vi "α粒子的能量损失.vi"() -> ()   [LabVIEW 2014]
panel:
  out "当前放射源":string(combo) caption="放射源"
  in  "放大倍数":dbl min=0.0 max=2.0
  in  "按钮_提示":bool caption="提示"
  in  "按钮_退出":bool caption="退出"
  out "是否真空":bool
  out "信号输出":bool
  out "是否放置吸收片":bool
  out "是否放置放射源":bool
  in  "数组_电压数据名":string[](array[string])
  in  "选项卡_实验内容":T1(tab)
  in  "按钮_恢复仪器初始状态 2":bool
  in  "选项卡控件_实验步骤1":T2(tab)
  in  "选项卡控件_操作步骤1":enum32{"选项卡 1", "选项卡 2", "选项卡 3", "选项卡 4"}(tab)
  out "偏压输入指示":bool caption="偏压输入"
  out "信号输出指示":bool caption="信号输出"
  in  "按钮_抽取真空":bool
  in  "放射源":string(combo)
  in  "按钮_放置放射源":bool
  in  "按钮_开始测量":bool
  in  "按钮_加电压":bool
  out "电压表":i32(knob) scale=0.0..130.0
  in  "按钮_恢复仪器初始状态 3":bool
  in  "按钮_抽取真空 2":bool
  in  "选项卡控件 操作步骤3":enum32{"选项卡 1", "选项卡 2"}(tab)
  in  "选项卡控件_实验步骤2":T2(tab)
  out "信号输出指示 2":bool caption="信号输出"
  in  "放射源2":string(combo) caption="放射源"
  in  "按钮_加载高压":bool
  in  "按钮_开始测量2":bool
  in  "按钮_放置放射源2":bool
  out "电压表 2":i32(knob) caption="电压表" scale=0.0..200.0
  out "偏压输入指示 2":bool caption="偏压输入"
  in  "按钮_恢复仪器初始状态":bool
  in  "按钮_抽取真空 3":bool
  in  "选项卡控件 操作步骤2":enum32{"选项卡 1", "选项卡 2"}(tab)
  in  "选项卡控件_实验步骤3":T2(tab)
  out "信号输出指示 3":bool caption="信号输出"
  in  "吸收片种类":string(combo)
  in  "按钮_加载高压 2":bool
  in  "按钮_开始测量3":bool
  in  "按钮_放置吸收片":bool
  out "电压表 3":i32(knob) caption="电压表" scale=0.0..200.0
  out "偏压输入指示 3":bool caption="偏压输入"
  out "退出":bool
  # "实验：α粒子的能量损失"
  # "实验原理"
  # "实验仪器"
  # "实验步骤"
  # "实验原理"
  # "实验仪器"
  # "实验步骤"
  # "实验原理"
  # "实验仪器"
  # "实验步骤"
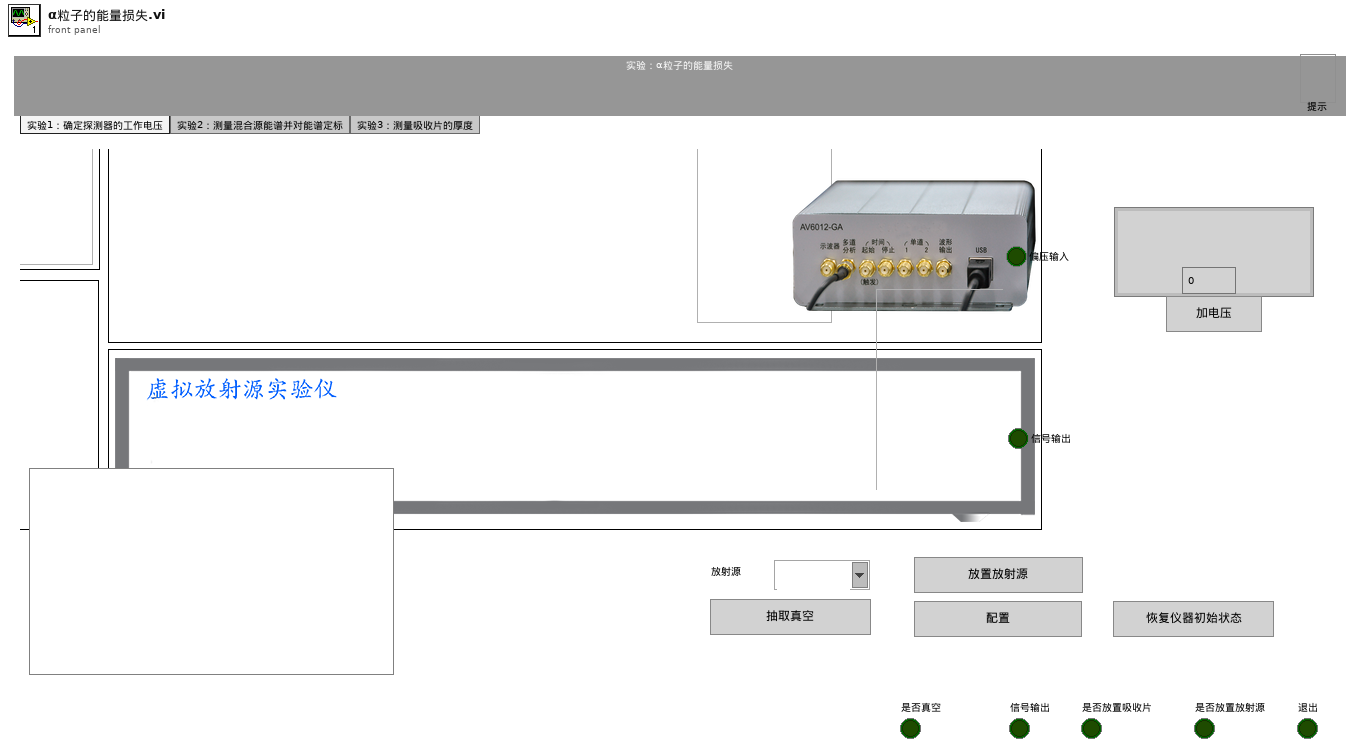
[diagram p1: front panel]
types:
  T1 = enum32{"实验1：确定探测器的工作电压", "实验2：测量混合源能谱并对能谱定标", "实验3：测量吸收片的厚度"}
  T2 = enum32{"选项卡 1", "选项卡 2", "选项卡 3", "选项卡 4", "选项卡 5", "选项卡 6", "选项卡 7", "选项卡 8", "选项卡 9", "选项卡 10", "选项卡 11"}
  T3 = enum8{"Enabled", "Disabled", "Disabled and Grayed Out"}
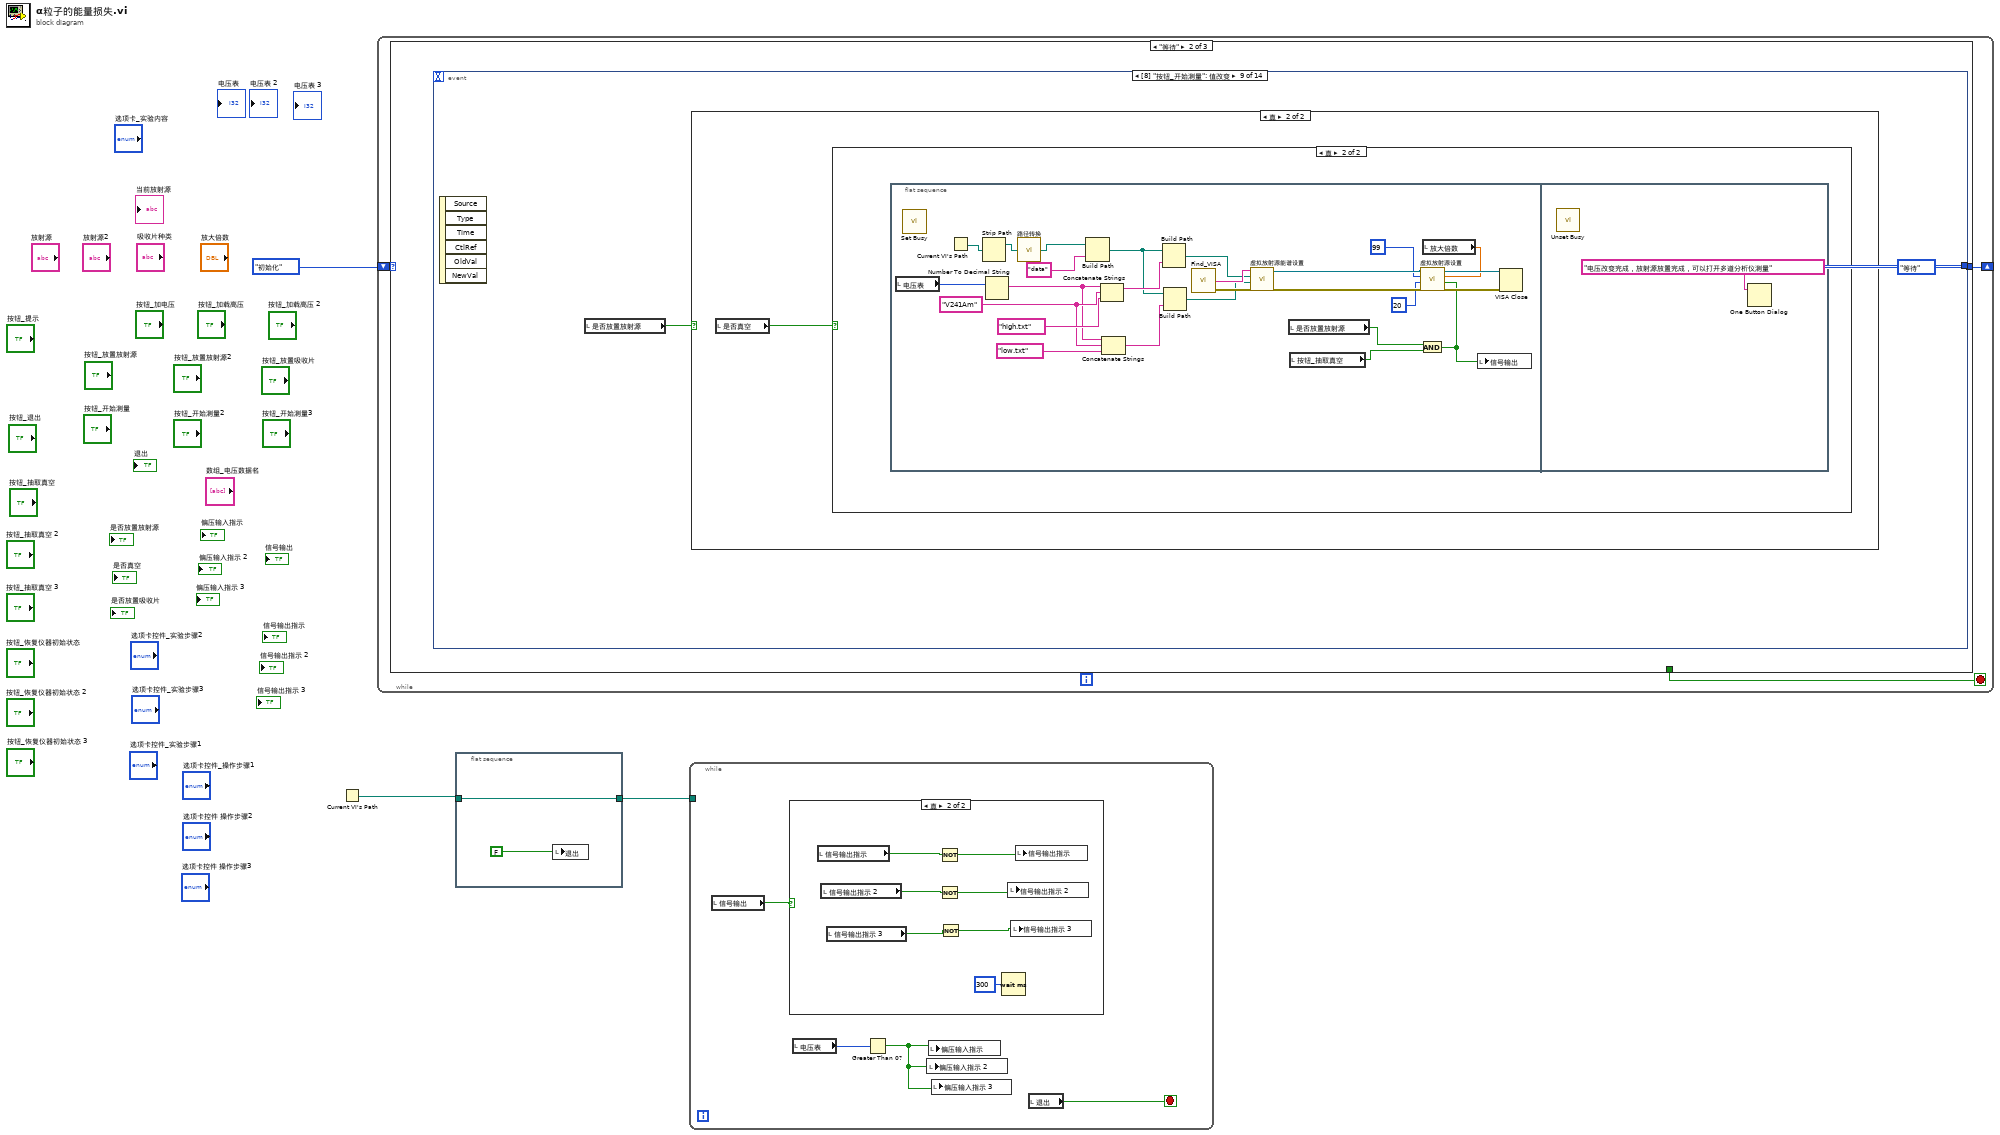
[diagram p0: block diagram]
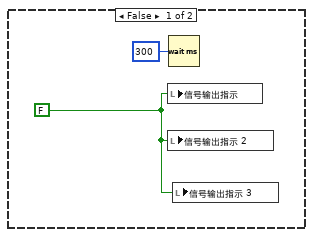
[diagram p2: hidden frame]
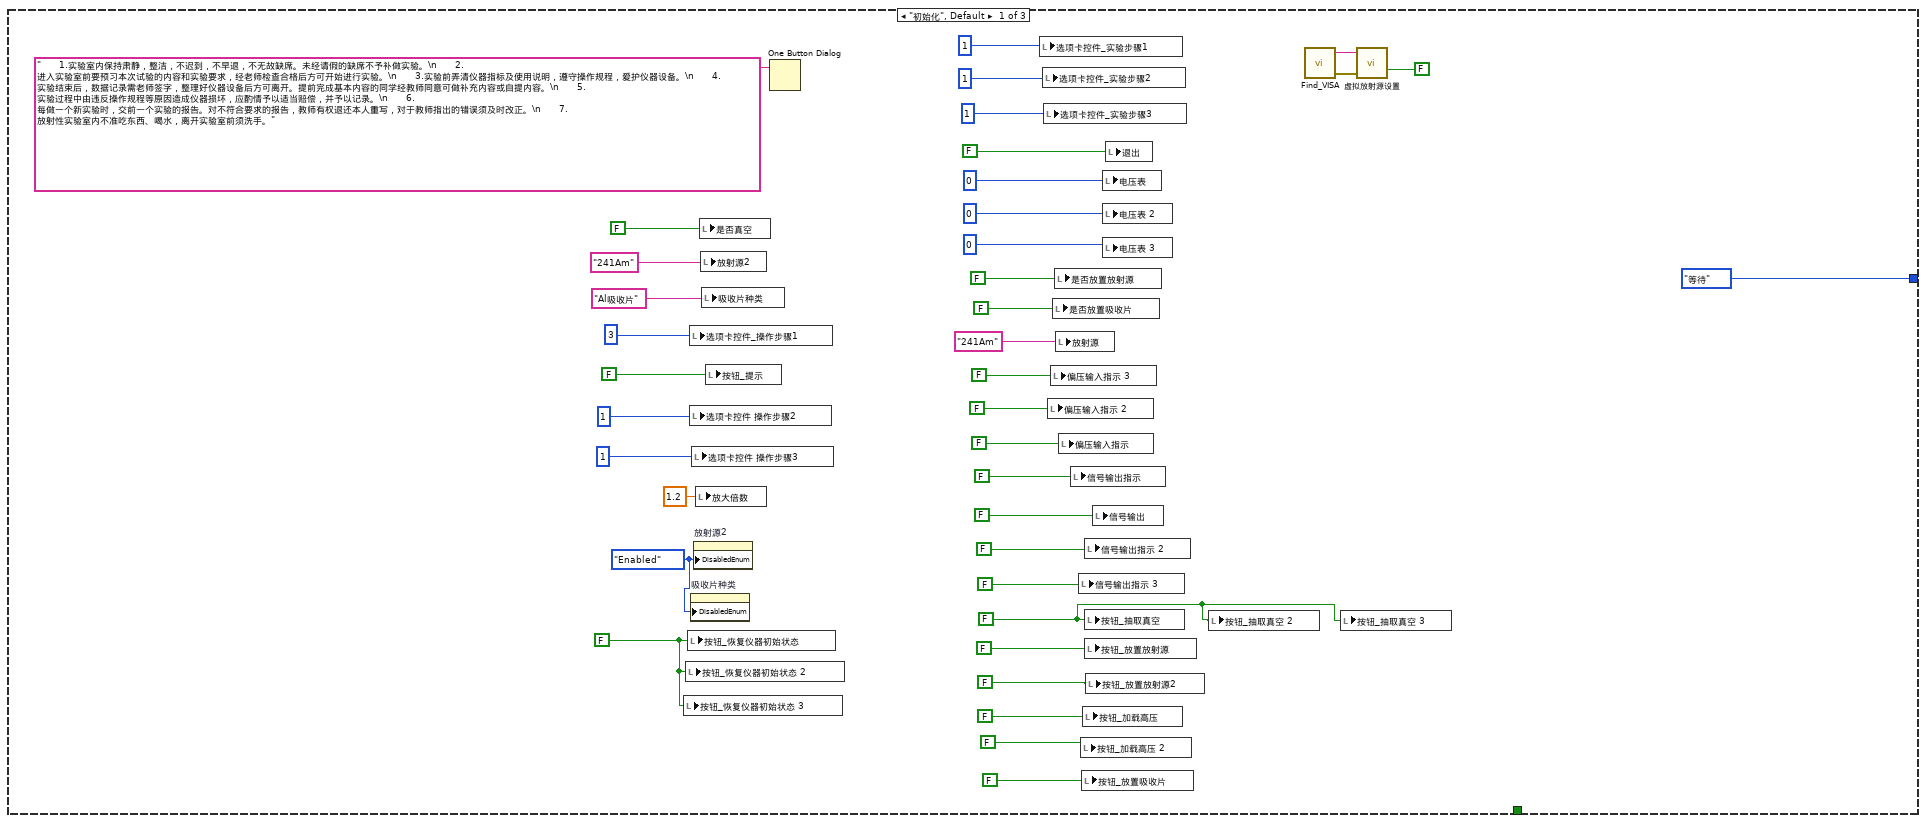
[diagram p3: hidden frame]
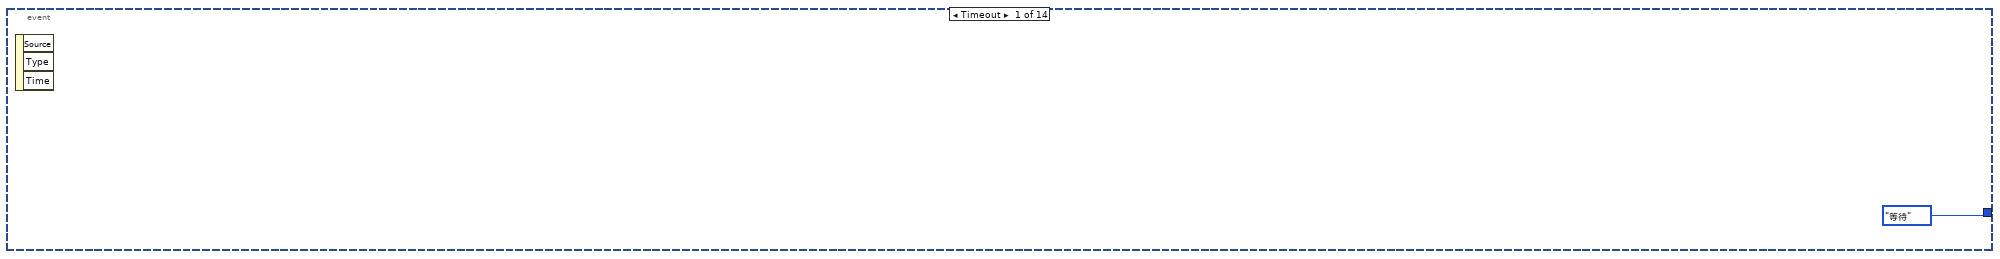
[diagram p4: hidden frame]
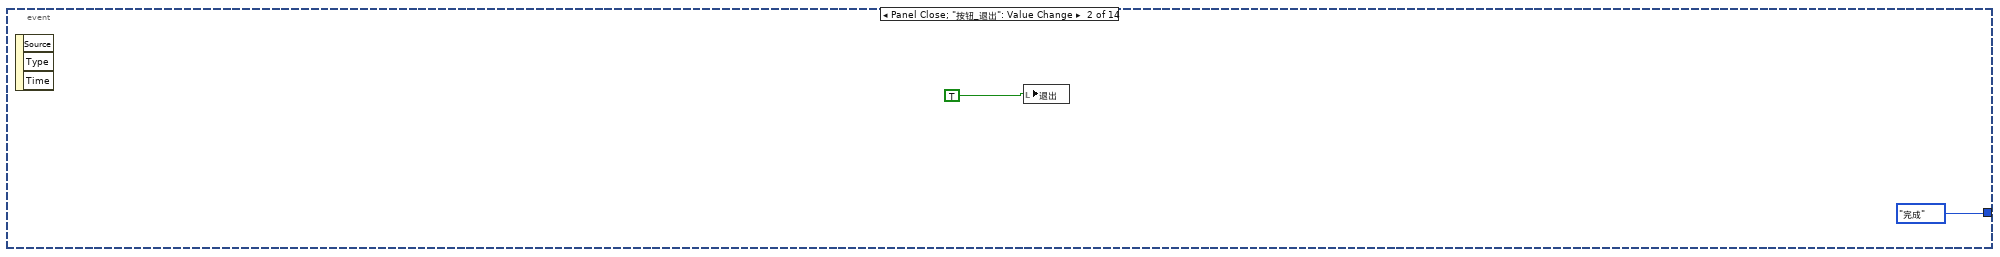
[diagram p5: hidden frame]
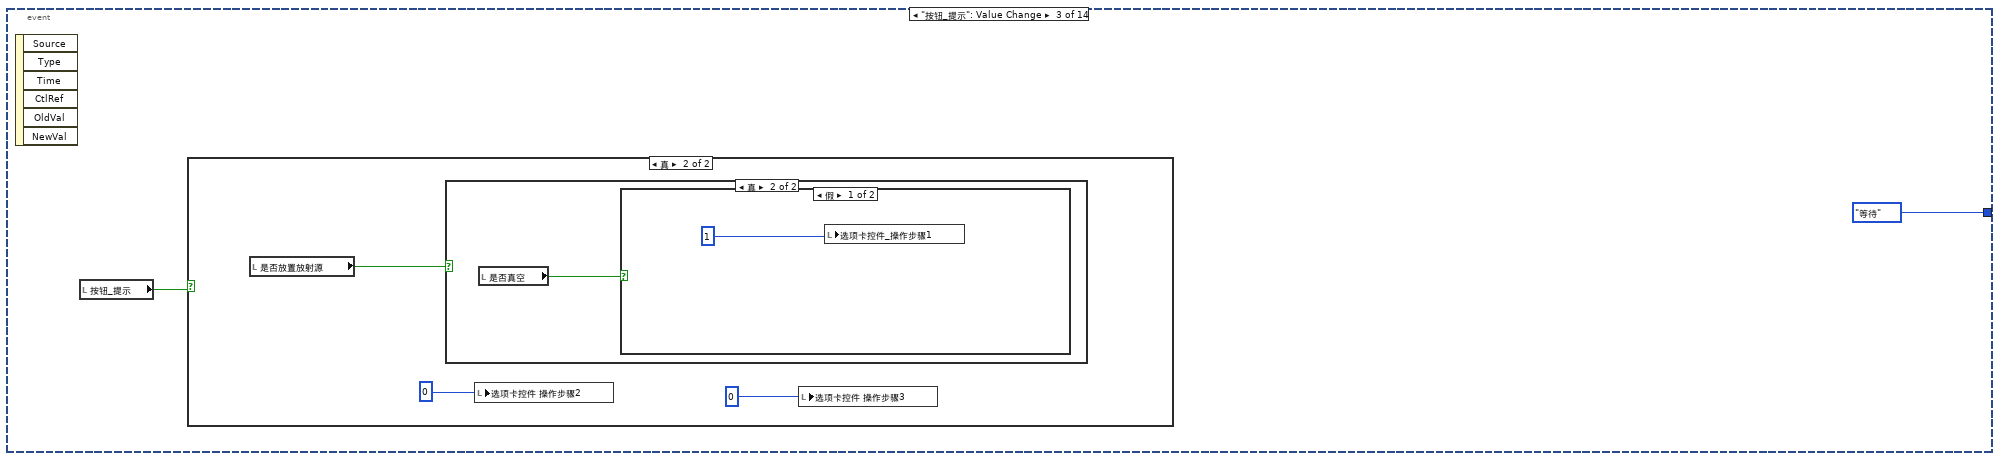
[diagram p6: hidden frame]
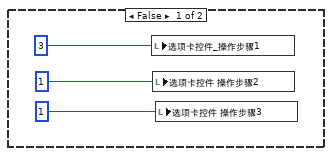
[diagram p7: hidden frame]
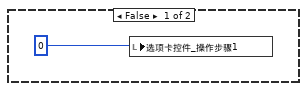
[diagram p8: hidden frame]
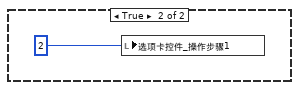
[diagram p9: hidden frame]
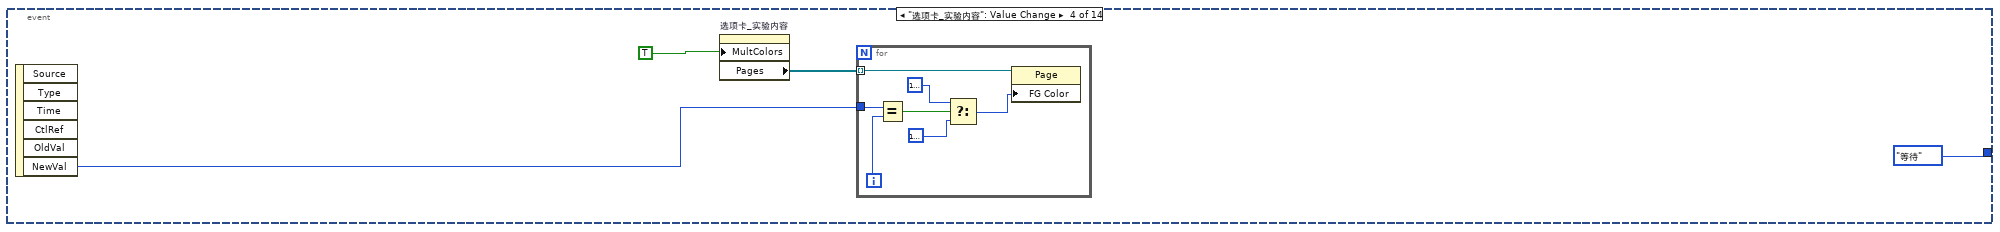
[diagram p10: hidden frame]
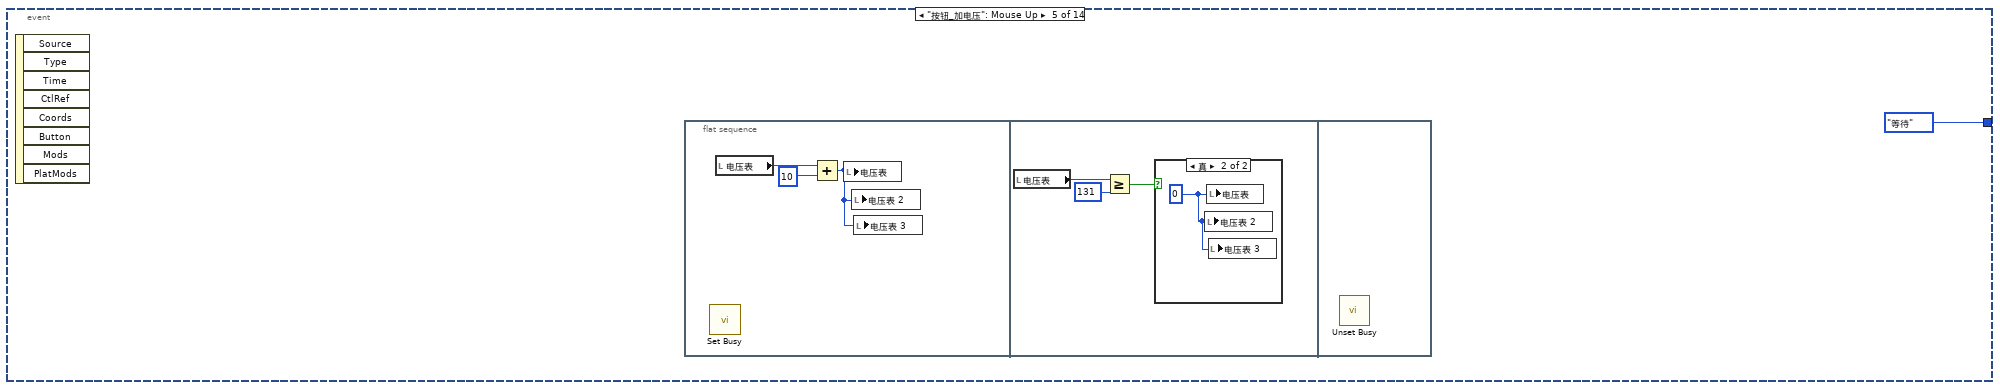
[diagram p11: hidden frame]
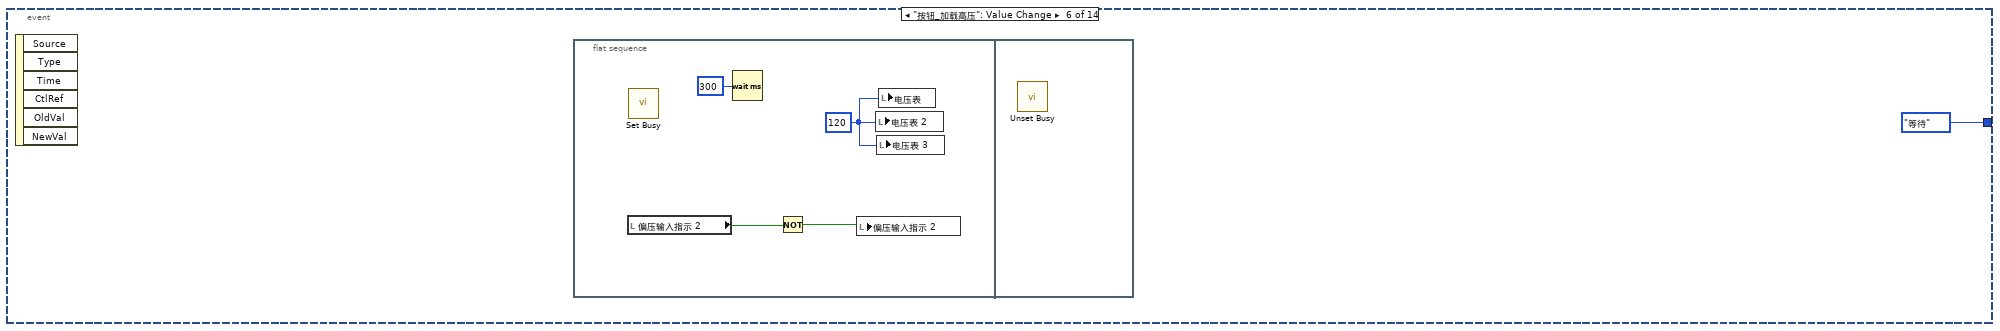
[diagram p13: hidden frame]
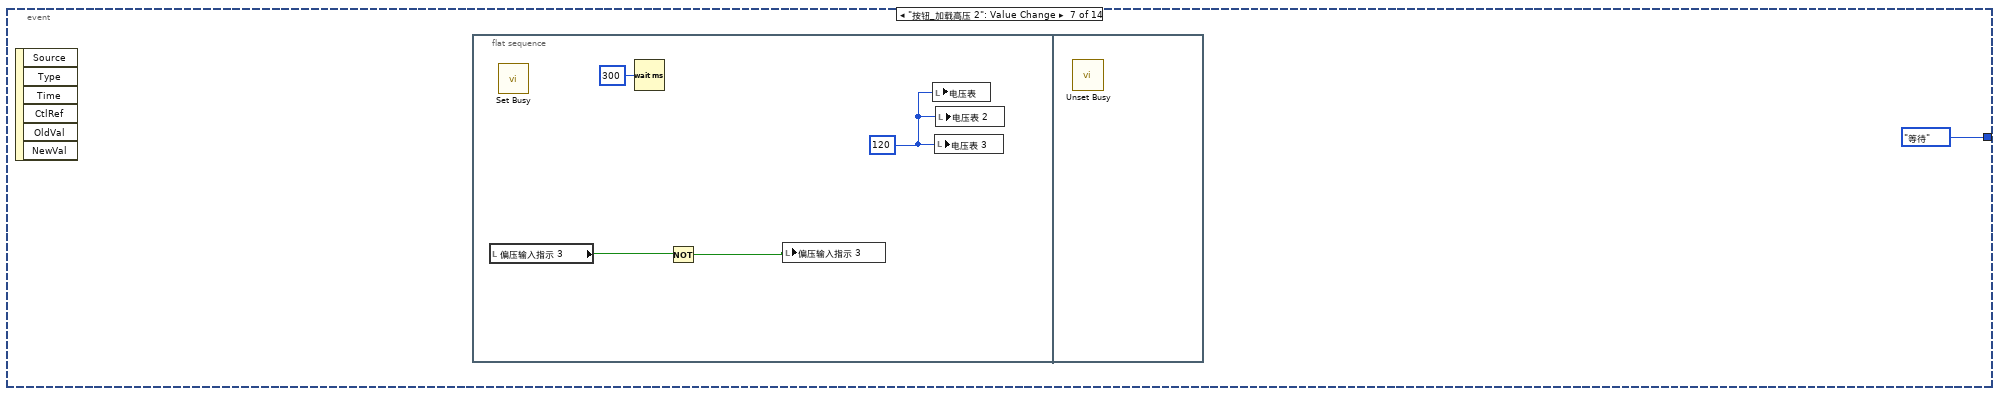
[diagram p14: hidden frame]
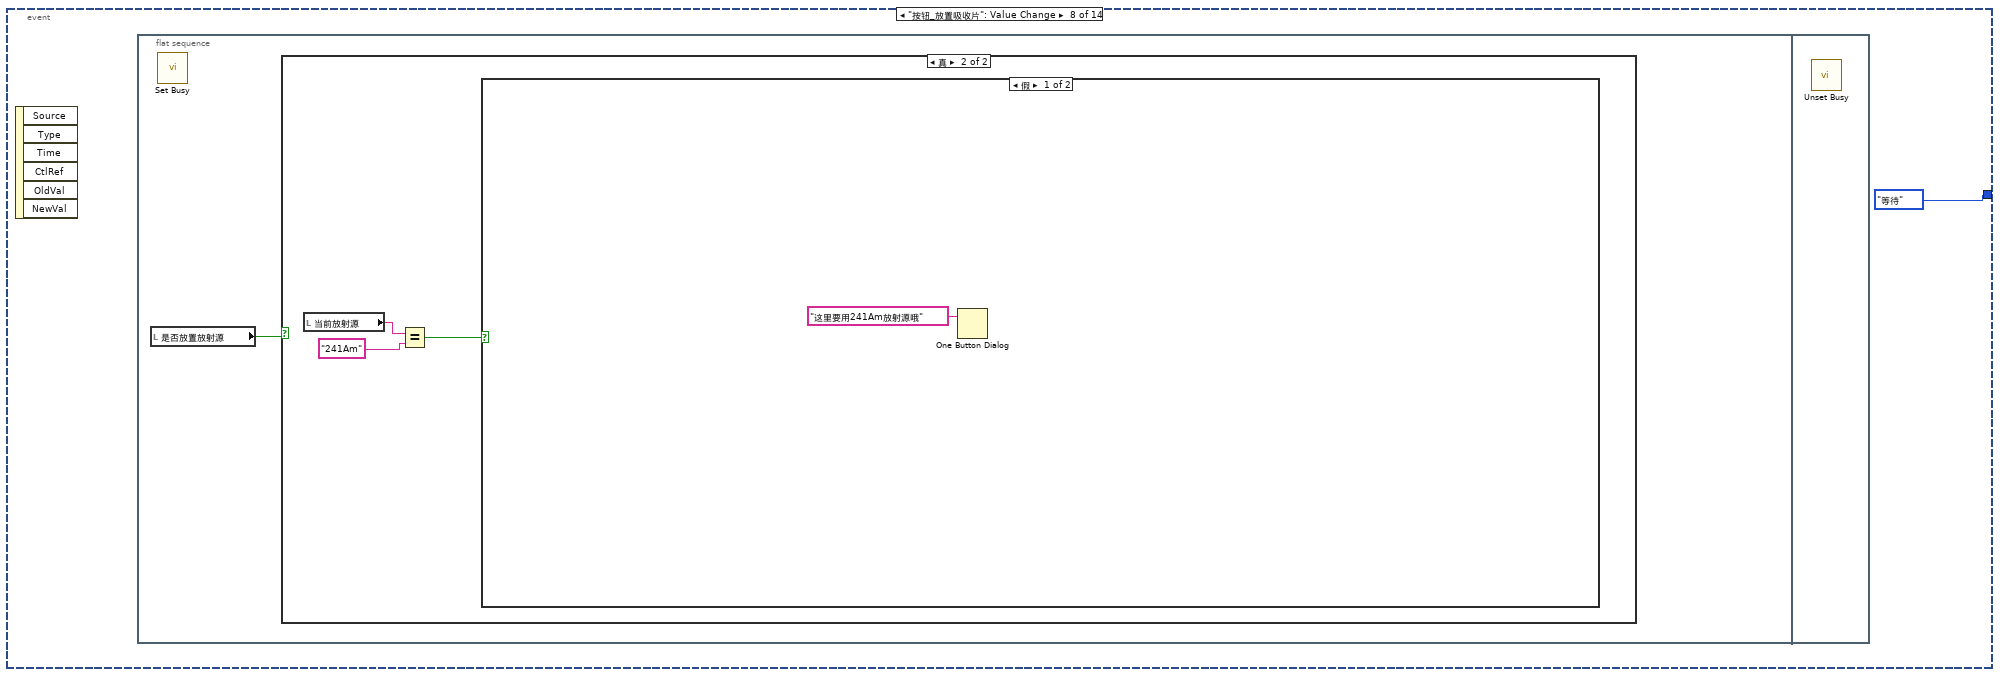
[diagram p15: hidden frame]
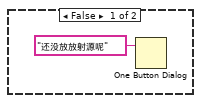
[diagram p16: hidden frame]
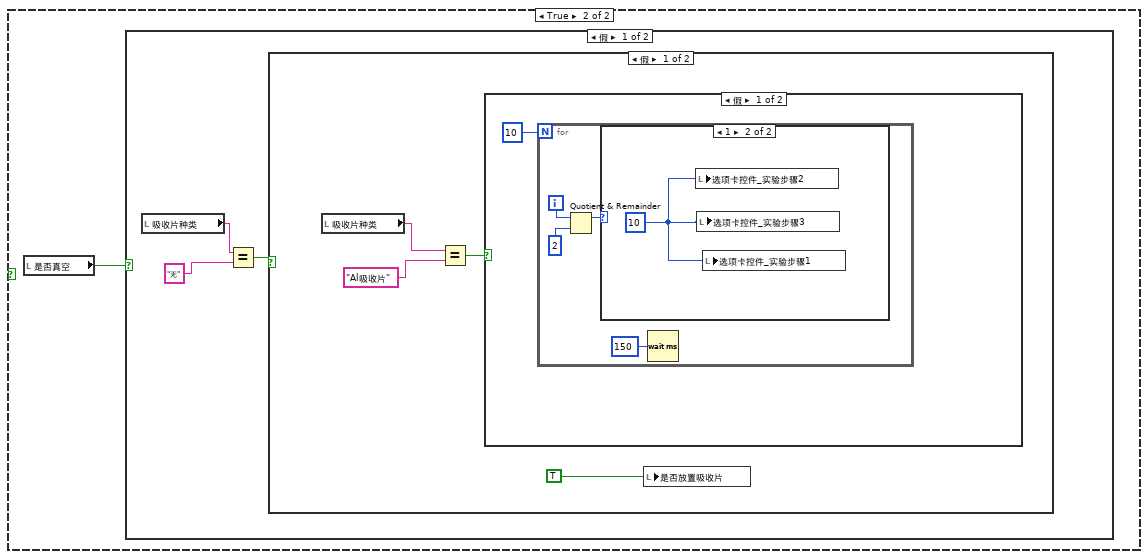
[diagram p17: hidden frame]
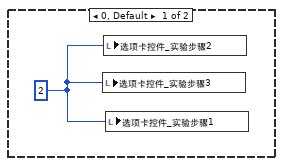
[diagram p18: hidden frame]
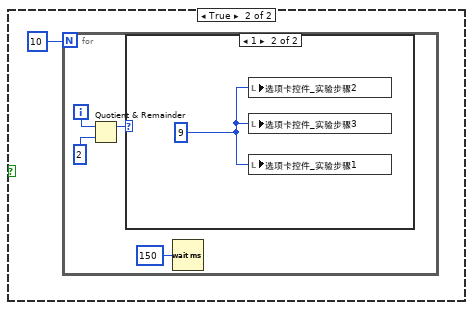
[diagram p19: hidden frame]
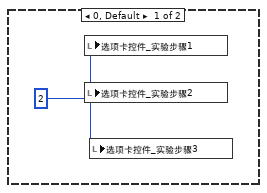
[diagram p20: hidden frame]
diagram:
  n1 = Current VI's Path() -> (path=w2:path)
  n2 = while {
    shift-right: [w5] -> _
    shift-left: enum16{"初始化", "等待", "完成"}."初始化" -> [w6]
    stop <- w4 stop-if-true
    n3 = case shown="\"等待\"" w6 {
      tunnel: [enum16{"初始化", "等待", "完成"}."等待" w45 enum16{"初始化", "等待", "完成"}."完成"] -> w5
      tunnel: [_ _ TRUE] -> w4
      frame "初始化", Default {
        w10 = FALSE ("按钮_恢复仪器初始状态")
        w11 = T3."Enabled" ("禁用")
        w12 = FALSE
        n4 = local write "按钮_恢复仪器初始状态 3"(w10) -> ()
        n5 = local write "按钮_恢复仪器初始状态 2"(w10) -> ()
        n6 = local write "按钮_恢复仪器初始状态"(w10) -> ()
        n7 = local write "选项卡控件_操作步骤1"(3) -> ()
        n8 = local write "选项卡控件 操作步骤2"(1) -> ()
        n9 = property on="吸收片种类" class="CmbBox"("DisabledEnum"=w11) -> ()  [unwired: 2 in, 2 out]
        n10 = local write "选项卡控件 操作步骤3"(1) -> ()
        n11 = property on="放射源2" class="CmbBox"("DisabledEnum"=w11) -> ()  [unwired: 2 in, 2 out]
        n12 = local write "放大倍数"(1.2 ("放大倍数")) -> ()
        n13 = local write "是否真空"(FALSE) -> ()
        n14 = local write "放射源2"("241Am") -> ()
        n15 = local write "吸收片种类"("Al吸收片") -> ()
        n16 = local write "按钮_提示"(FALSE) -> ()
        n17 = One Button Dialog(message="      1.实验室内保持肃静，整洁，不迟到，不早退，不无故缺席。未经请假的缺席不予补做实验。\n      2.进入实验室前要预习本次试验的内容和实验要求，经老师检查合格后方可开始进行实验。\n      3.实验前弄清仪器指标及使用说明，遵守操作规程，爱护仪器设备。\n      4.实验结束后，数据记录需老师签字，整理好仪器设备后方可离开。提前完成基本内容的同学经教师同意可做补充内容或自提内容。\n      5.实验过程中由违反操作规程等原因造成仪器损坏，应酌情予以适当赔偿，并予以记录。\n      6.每做一个新实验时，交前一个实验的报告。对不符合要求的报告，教师有权退还本人重写，对于教师指出的错误须及时改正。\n      7.放射性实验室内不准吃东西、喝水，离开实验室前须洗手。" ("消息")) -> ()  [unwired: 1 in, 1 out]
        n18 = local write "选项卡控件_实验步骤1"(1) -> ()
        n19 = local write "选项卡控件_实验步骤2"(1) -> ()
        n20 = local write "选项卡控件_实验步骤3"(1) -> ()
        n21 = local write "偏压输入指示 2"(FALSE) -> ()
        n22 = local write "偏压输入指示 3"(FALSE) -> ()
        n23 = local write "是否放置吸收片"(FALSE) -> ()
        n24 = local write "是否放置放射源"(FALSE) -> ()
        n25 = local write "放射源"("241Am") -> ()
        n26 = local write "偏压输入指示"(FALSE) -> ()
        n27 = local write "信号输出指示"(FALSE) -> ()
        n28 = local write "信号输出指示 3"(FALSE) -> ()
        n29 = local write "按钮_加载高压 2"(FALSE) -> ()
        n30 = local write "按钮_放置吸收片"(FALSE) -> ()
        n31 = local write "按钮_加载高压"(FALSE) -> ()
        n32 = local write "信号输出指示 2"(FALSE) -> ()
        n33 = local write "按钮_抽取真空"(w12) -> ()
        n34 = local write "按钮_放置放射源"(FALSE) -> ()
        n35 = local write "按钮_放置放射源2"(FALSE) -> ()
        n36 = local write "信号输出"(FALSE) -> ()
        n37 = local write "电压表"(0) -> ()
        n38 = local write "电压表 2"(0) -> ()
        n39 = local write "电压表 3"(0) -> ()
        n40 = local write "退出"(FALSE) -> ()
        n41 = local write "按钮_抽取真空 2"(w12) -> ()
        n42 = call "Find_VISA.vi"() -> ("错误输出"=w8:errorcluster, "多道VISA"=w9:string)  [unwired: 3 in, 1 out]
        n43 = local write "按钮_抽取真空 3"(w12) -> ()
        n44 = call "虚拟放射源设置.vi"("信号输出"=FALSE, "错误输入（无错误）"=w8, "VISA资源名称"=w9) -> ()  [unwired: 3 in, 2 out]
      }
      frame "等待" {
        n45 = event shown="[8] \"按钮_开始测量\": 值改变" {
          selector: _ -> [_ _ _ _ _ _ _ _ _ _ _ _ _ _]
          dyn-events: _ -> [_ _ _ _ _ _ _ _ _ _ _ _ _ _]
          timeout: _ -> [_ _ _ _ _ _ _ _ _ _ _ _ _ _]
          tunnel: [enum16{"初始化", "等待", "完成"}."等待" enum16{"初始化", "等待", "完成"}."完成" enum16{"初始化", "等待", "完成"}."等待" enum16{"初始化", "等待", "完成"}."等待" enum16{"初始化", "等待", "完成"}."等待" enum16{"初始化", "等待", "完成"}."等待" enum16{"初始化", "等待", "完成"}."等待" enum16{"初始化", "等待", "完成"}."等待" enum16{"初始化", "等待", "完成"}."等待" enum16{"初始化", "等待", "完成"}."等待" enum16{"初始化", "等待", "完成"}."等待" enum16{"初始化", "等待", "完成"}."等待" enum16{"初始化", "等待", "完成"}."等待" enum16{"初始化", "等待", "完成"}."等待"] -> w45
          event Timeout {
            n46 = event-data() -> ()  [unwired: 1 in, 3 out]
          }
          event Panel Close; "按钮_退出": Value Change {
            n47 = event-data() -> ()  [unwired: 1 in, 3 out]
            n48 = local write "退出"(TRUE) -> ()
          }
          event "按钮_提示": Value Change {
            n49 = event-data() -> ()  [unwired: 1 in, 6 out]
            n50 = local read "按钮_提示"() -> (w49:bool)
            n51 = case shown="真" w49 {
              frame False {
                n52 = local write "选项卡控件_操作步骤1"(3) -> ()
                n53 = local write "选项卡控件 操作步骤2"(1) -> ()
                n54 = local write "选项卡控件 操作步骤3"(1) -> ()
              }
              frame True {
                n55 = local read "是否放置放射源"() -> (w56:bool)
                n56 = case shown="真" w56 {
                  frame False {
                    n57 = local write "选项卡控件_操作步骤1"(0) -> ()
                  }
                  frame True {
                    n58 = local read "是否真空"() -> (w58:bool)
                    n59 = case shown="假" w58 {
                      frame False {
                        n60 = local write "选项卡控件_操作步骤1"(1) -> ()
                      }
                      frame True {
                        n61 = local write "选项卡控件_操作步骤1"(2) -> ()
                      }
                    }
                  }
                }
                n62 = local write "选项卡控件 操作步骤2"(0) -> ()
                n63 = local write "选项卡控件 操作步骤3"(0) -> ()
              }
            }
          }
          event "选项卡_实验内容": Value Change {
            n64 = event-data() -> ("NewVal"=w62:T1)  [unwired: 1 in, 5 out]
            n65 = property on="选项卡_实验内容" class="TabCtl (严格)"("MultColors"=TRUE) -> ("Pages"=w63:refnum<vi>[])  [unwired: 2 in, 2 out]
            n66 = for {
              tunnel: w63 -> [w71] mode=indexing
              tunnel: w62 -> [w65]
              i -> [w66]
              n67 = Equal?(x=w65, y=w66) -> (x = y?=w67:bool)
              n68 = Select(t=u32 16777216, s=w67, f=u32 16777226) -> (s? t:f=w70:u32)
              n69 = property class="Page"(reference=w71, "FG Color"=w70) -> ()  [unwired: 1 in, 2 out]
            }
          }
          event "按钮_加电压": Mouse Up {
            n70 = event-data() -> ()  [unwired: 1 in, 8 out]
            n71 = flat-sequence {
              frame #0 {
                n72 = call <vilib>:"Set Busy.vi"() -> ()  [unwired: 10 in, 2 out]
                n73 = local read "电压表"() -> (w74:i32)
                n74 = Add(x=w74, y=10) -> (x+y=w73:i32)
                n75 = local write "电压表"(w73) -> ()
                n76 = local write "电压表 2"(w73) -> ()
                n77 = local write "电压表 3"(w73) -> ()
              }
              frame #1 {
                n78 = local read "电压表"() -> (w78:i32)
                n79 = Greater Or Equal?(x=w78, y=131) -> (x >= y?=w77:bool)
                n80 = case shown="真" w77 {
                  frame False {
                  }
                  frame True {
                    w79 = 0
                    n81 = local write "电压表 2"(w79) -> ()
                    n82 = local write "电压表"(w79) -> ()
                    n83 = local write "电压表 3"(w79) -> ()
                  }
                }
              }
              frame #2 {
                n84 = call <vilib>:"Unset Busy.vi"() -> ()  [unwired: 11 in, 1 out]
              }
            }
          }
          event "按钮_加载高压": Value Change {
            n85 = event-data() -> ()  [unwired: 1 in, 6 out]
            n86 = flat-sequence {
              frame #0 {
                w82 = 120
                n87 = local read "偏压输入指示 2"() -> (w84:bool)
                n88 = call <vilib>:"Set Busy.vi"() -> ()  [unwired: 10 in, 2 out]
                n89 = Wait (ms)(milliseconds to wait=u32 300 ("等待时间（毫秒）")) -> ()  [unwired: 1 out]
                n90 = Not(x=w84) -> (.not. x?=w83:bool)
                n91 = local write "偏压输入指示 2"(w83) -> ()
                n92 = local write "电压表 2"(w82) -> ()
                n93 = local write "电压表 3"(w82) -> ()
                n94 = local write "电压表"(w82) -> ()
              }
              frame #1 {
                n95 = call <vilib>:"Unset Busy.vi"() -> ()  [unwired: 11 in, 1 out]
              }
            }
          }
          event "按钮_加载高压 2": Value Change {
            n96 = event-data() -> ()  [unwired: 1 in, 6 out]
            n97 = flat-sequence {
              frame #0 {
                w87 = 120
                n98 = local read "偏压输入指示 3"() -> (w89:bool)
                n99 = call <vilib>:"Set Busy.vi"() -> ()  [unwired: 10 in, 2 out]
                n100 = Wait (ms)(milliseconds to wait=u32 300 ("等待时间（毫秒）")) -> ()  [unwired: 1 out]
                n101 = Not(x=w89) -> (.not. x?=w88:bool)
                n102 = local write "偏压输入指示 3"(w88) -> ()
                n103 = local write "电压表"(w87) -> ()
                n104 = local write "电压表 3"(w87) -> ()
                n105 = local write "电压表 2"(w87) -> ()
              }
              frame #1 {
                n106 = call <vilib>:"Unset Busy.vi"() -> ()  [unwired: 11 in, 1 out]
              }
            }
          }
          event "按钮_放置吸收片": Value Change {
            n107 = event-data() -> ()  [unwired: 1 in, 6 out]
            n108 = flat-sequence {
              frame #0 {
                n109 = local read "是否放置放射源"() -> (w91:bool)
                n110 = call <vilib>:"Set Busy.vi"() -> ()  [unwired: 10 in, 2 out]
                n111 = case shown="真" w91 {
                  frame False {
                    n112 = One Button Dialog(message="还没放放射源呢" ("消息")) -> ()  [unwired: 1 in, 1 out]
                  }
                  frame True {
                    n113 = local read "当前放射源"() -> (w94:string)
                    n114 = Equal?(x=w94, y="241Am") -> (x = y?=w93:bool)
                    n115 = case shown="假" w93 {
                      frame False {
                        n116 = One Button Dialog(message="这里要用241Am放射源哦" ("消息")) -> ()  [unwired: 1 in, 1 out]
                      }
                      frame True {
                        n117 = local read "是否真空"() -> (w97:bool)
                        n118 = case shown="假" w97 {
                          frame False {
                            n119 = local read "吸收片种类"() -> (w100:string)
                            n120 = Equal?(x=w100, y="无") -> (x = y?=w98:bool)
                            n121 = case shown="假" w98 {
                              frame False {
                                n122 = local read "吸收片种类"() -> (w104:string)
                                n123 = Equal?(x=w104, y="Al吸收片") -> (x = y?=w102:bool)
                                n124 = case shown="假" w102 {
                                frame False {
                                n125 = for {
                                N: 10 -> [_]
                                i -> [w107]
                                n126 = Quotient & Remainder(x=w107, y=2) -> (x-y*floor(x/y)=w108:i32)  [unwired: 1 out]
                                n127 = case shown="1" w108 {
                                frame 0, Default {
                                w110 = 2
                                n128 = local write "选项卡控件_实验步骤3"(w110) -> ()
                                n129 = local write "选项卡控件_实验步骤2"(w110) -> ()
                                n130 = local write "选项卡控件_实验步骤1"(w110) -> ()
                                }
                                frame 1 {
                                w111 = 10
                                n131 = local write "选项卡控件_实验步骤2"(w111) -> ()
                                n132 = local write "选项卡控件_实验步骤3"(w111) -> ()
                                n133 = local write "选项卡控件_实验步骤1"(w111) -> ()
                                }
                                }
                                n134 = Wait (ms)(milliseconds to wait=u32 150 ("等待时间（毫秒）")) -> ()  [unwired: 1 out]
                                }
                                }
                                frame True {
                                n135 = for {
                                N: 10 -> [_]
                                i -> [w114]
                                n136 = Quotient & Remainder(x=w114, y=2) -> (x-y*floor(x/y)=w115:i32)  [unwired: 1 out]
                                n137 = case shown="1" w115 {
                                frame 0, Default {
                                w117 = 2
                                n138 = local write "选项卡控件_实验步骤1"(w117) -> ()
                                n139 = local write "选项卡控件_实验步骤2"(w117) -> ()
                                n140 = local write "选项卡控件_实验步骤3"(w117) -> ()
                                }
                                frame 1 {
                                w118 = 9
                                n141 = local write "选项卡控件_实验步骤2"(w118) -> ()
                                n142 = local write "选项卡控件_实验步骤3"(w118) -> ()
                                n143 = local write "选项卡控件_实验步骤1"(w118) -> ()
                                }
                                }
                                n144 = Wait (ms)(milliseconds to wait=u32 150 ("等待时间（毫秒）")) -> ()  [unwired: 1 out]
                                }
                                }
                                }
                                n145 = local write "是否放置吸收片"(TRUE) -> ()
                              }
                              frame True {
                                w120 = 2
                                n146 = local write "选项卡控件_实验步骤1"(w120) -> ()
                                n147 = local write "选项卡控件_实验步骤3"(w120) -> ()
                                n148 = local write "是否放置吸收片"(FALSE ("是否放置吸收片")) -> ()
                                n149 = local write "选项卡控件_实验步骤2"(w120) -> ()
                              }
                            }
                          }
                          frame True {
                            n150 = One Button Dialog(message="只有先放气才能打开真空室" ("消息")) -> ()  [unwired: 1 in, 1 out]
                          }
                        }
                      }
                    }
                  }
                }
              }
              frame #1 {
                n151 = call <vilib>:"Unset Busy.vi"() -> ()  [unwired: 11 in, 1 out]
              }
            }
          }
          event "按钮_开始测量": Value Change {
            n152 = event-data() -> ()  [unwired: 1 in, 6 out]
            n153 = local read "是否放置放射源"() -> (w122:bool)
            n154 = case shown="真" w122 {
              frame False {
                n155 = One Button Dialog(message="还没放放射源，会没有信号的" ("消息")) -> ()  [unwired: 1 in, 1 out]
              }
              frame True {
                n156 = local read "是否真空"() -> (w125:bool)
                n157 = case shown="真" w125 {
                  frame False {
                    n158 = One Button Dialog(message="还没抽真空，测出来的数据不准确的" ("消息")) -> ()  [unwired: 1 in, 1 out]
                  }
                  frame True {
                    n159 = flat-sequence {
                      frame #0 {
                        w141 = "V241Am"
                        n160 = local read "电压表"() -> (w142:i32)
                        n161 = call <vilib>:"Set Busy.vi"() -> ()  [unwired: 10 in, 2 out]
                        n162 = Current VI's Path() -> (path=w129:path)
                        n163 = Strip Path(path=w129) -> (stripped path=w128:path)  [unwired: 1 out]
                        n164 = Number To Decimal String(number=w142) -> (decimal integer string=w140:string)  [unwired: 1 in]
                        n165 = call "路径转换.vi"("input path"=w128) -> ("output path"=w127:path)
                        n166 = Build Path(base path=w127, name or relative path="data") -> (appended path=w143:path)
                        n167 = Concatenate Strings(w140, w141, "high.txt") -> (w149:string)
                        n168 = Concatenate Strings(w140, w141, "low.txt") -> (w152:string)
                        n169 = Build Path(base path=w143, name or relative path=w149) -> (appended path=w144:path)
                        n170 = Build Path(base path=w143, name or relative path=w152) -> (appended path=w145:path)
                        n171 = call "Find_VISA.vi"() -> ("错误输出"=w147:errorcluster, "虚拟放射源VISA"=w146:string)  [unwired: 3 in, 1 out]
                        n172 = call "虚拟放射源能谱设置.vi"("错误输入（无错误）"=w147, "低位数据路径"=w145, "高位数据路径"=w144, "VISA资源名称"=w146) -> ("错误输出"=w136:errorcluster, "VISA资源名称输出"=w138:refnum<visa-resource-name>)
                        n173 = local read "是否放置放射源"() -> (w139:bool)
                        n174 = local read "按钮_抽取真空"() -> (w130:bool)
                        n175 = And(x=w139, y=w130) -> (x .and. y?=w131:bool)
                        n176 = local read "放大倍数"() -> (w132:dbl)
                        n177 = call "虚拟放射源设置.vi"("信号输出"=w131, "放大倍数"=w132, "错误输入（无错误）"=w136, "最小时间间隔"=u16 20, "计数率"=99, "VISA资源名称"=w138) -> ("错误输出"=w135:errorcluster, "VISA资源名称输出"=w137:refnum<visa-resource-name>)
                        n178 = local write "信号输出"(w131) -> ()
                        n179 = VISA Close(VISA resource name=w137, error in (no error)=w135) -> ()  [unwired: 1 out]
                      }
                      frame #1 {
                        n180 = call <vilib>:"Unset Busy.vi"() -> ()  [unwired: 11 in, 1 out]
                        n181 = One Button Dialog(message="电压改变完成，放射源放置完成，可以打开多道分析仪测量") -> ()  [unwired: 1 in, 1 out]
                      }
                    }
                  }
                }
              }
            }
          }
          event "按钮_放置放射源2", "按钮_放置放射源": Value Change {
            n182 = event-data() -> ()  [unwired: 1 in, 6 out]
            n183 = flat-sequence {
              frame #0 {
                n184 = local read "是否放置吸收片"() -> (w157:bool)
                n185 = call <vilib>:"Set Busy.vi"() -> ()  [unwired: 10 in, 2 out]
                n186 = case shown="假" w157 {
                  frame False {
                    n187 = local read "是否放置放射源"() -> (w159:bool)
                    n188 = local read "是否真空"() -> (w160:bool)
                    n189 = Not Or(1:w160, 2:w159) -> (0:w158:bool)
                    n190 = case shown="假" w158 {
                      frame False {
                        n191 = local read "是否真空"() -> (w161:bool)
                        n192 = case shown="假" w161 {
                          frame False {
                            w165 = FALSE ("按钮_放置放射源")
                            n193 = local read "当前放射源"() -> (w168:string)
                            n194 = Equal?(x=w168, y="239Pu") -> (x = y?=w163:bool)
                            n195 = local write "是否放置放射源"(FALSE ("是否放置放射源")) -> ()
                            n196 = case shown="真" w163 {
                              frame False {
                                n197 = for {
                                N: 10 -> [_]
                                i -> [w171]
                                n198 = Quotient & Remainder(x=w171, y=2) -> (x-y*floor(x/y)=w172:i32)  [unwired: 1 out]
                                n199 = case shown="1" w172 {
                                frame 0, Default {
                                w174 = 2
                                n200 = local write "选项卡控件_实验步骤2"(w174) -> ()
                                n201 = local write "选项卡控件_实验步骤3"(w174) -> ()
                                n202 = local write "选项卡控件_实验步骤1"(w174) -> ()
                                }
                                frame 1 {
                                w175 = 1
                                n203 = local write "选项卡控件_实验步骤3"(w175) -> ()
                                n204 = local write "选项卡控件_实验步骤2"(w175) -> ()
                                n205 = local write "选项卡控件_实验步骤1"(w175) -> ()
                                }
                                }
                                n206 = Wait (ms)(milliseconds to wait=u32 150 ("等待时间（毫秒）")) -> ()  [unwired: 1 out]
                                }
                              }
                              frame True {
                                n207 = for {
                                N: 10 -> [_]
                                i -> [w178]
                                n208 = Quotient & Remainder(x=w178, y=2) -> (x-y*floor(x/y)=w179:i32)  [unwired: 1 out]
                                n209 = case shown="0, 默认" w179 {
                                frame 0, Default {
                                w181 = 8
                                n210 = local write "选项卡控件_实验步骤3"(w181) -> ()
                                n211 = local write "选项卡控件_实验步骤2"(w181) -> ()
                                n212 = local write "选项卡控件_实验步骤1"(w181) -> ()
                                }
                                frame 1 {
                                w182 = 1
                                n213 = local write "选项卡控件_实验步骤3"(w182) -> ()
                                n214 = local write "选项卡控件_实验步骤1"(w182) -> ()
                                n215 = local write "选项卡控件_实验步骤2"(w182) -> ()
                                }
                                }
                                n216 = Wait (ms)(milliseconds to wait=u32 150 ("等待时间（毫秒）")) -> ()  [unwired: 1 out]
                                }
                              }
                            }
                            n217 = property on="放射源2" class="CmbBox"("DisabledEnum"=T3."Enabled" ("禁用")) -> ()  [unwired: 2 in, 2 out]
                            n218 = local write "按钮_放置放射源2"(w165) -> ()
                            n219 = local write "按钮_放置放射源"(w165) -> ()
                            n220 = local write "放射源"("241Am" ("放射源")) -> ()
                          }
                          frame True {
                            w183 = TRUE ("按钮_放置放射源2")
                            n221 = local write "按钮_放置放射源2"(w183) -> ()
                            n222 = local write "按钮_放置放射源"(w183) -> ()
                            n223 = One Button Dialog(message="只有先放气才能打开真空室" ("消息")) -> ()  [unwired: 1 in, 1 out]
                          }
                        }
                      }
                      frame True {
                        w191 = TRUE
                        n224 = local read "放射源2"() -> (w193:string)
                        n225 = local read "选项卡_实验内容"() -> (w189:T1)
                        n226 = property on="放射源2" class="CmbBox"("DisabledEnum"=T3."Disabled and Grayed Out" ("禁用")) -> ()  [unwired: 2 in, 2 out]
                        n227 = Equal?(x=w193, y="239Pu") -> (x = y?=w187:bool)
                        n228 = Equal?(x=w189, y=1) -> (x = y?=w186:bool)
                        n229 = And(x=w187, y=w186) -> (x .and. y?=w185:bool)
                        n230 = case shown="假" w185 {
                          frame False {
                            n231 = for {
                              N: 10 -> [_]
                              i -> [w197]
                              n232 = Quotient & Remainder(x=w197, y=2) -> (x-y*floor(x/y)=w198:i32)  [unwired: 1 out]
                              n233 = case shown="0, 默认" w198 {
                                frame 0, Default {
                                w200 = 1
                                n234 = local write "选项卡控件_实验步骤1"(w200) -> ()
                                n235 = local write "选项卡控件_实验步骤3"(w200) -> ()
                                n236 = local write "选项卡控件_实验步骤2"(w200) -> ()
                                }
                                frame 1 {
                                w201 = 2
                                n237 = local write "选项卡控件_实验步骤1"(w201) -> ()
                                n238 = local write "选项卡控件_实验步骤2"(w201) -> ()
                                n239 = local write "选项卡控件_实验步骤3"(w201) -> ()
                                }
                              }
                              n240 = Wait (ms)(milliseconds to wait=u32 150 ("等待时间（毫秒）")) -> ()  [unwired: 1 out]
                            }
                            n241 = local write "当前放射源"("241Am") -> ()
                          }
                          frame True {
                            w202 = "239Pu"
                            n242 = for {
                              N: 10 -> [_]
                              i -> [w205]
                              n243 = Quotient & Remainder(x=w205, y=2) -> (x-y*floor(x/y)=w206:i32)  [unwired: 1 out]
                              n244 = case shown="1" w206 {
                                frame 0, Default {
                                w208 = 1
                                n245 = local write "选项卡控件_实验步骤2"(w208) -> ()
                                n246 = local write "选项卡控件_实验步骤3"(w208) -> ()
                                n247 = local write "选项卡控件_实验步骤1"(w208) -> ()
                                }
                                frame 1 {
                                w209 = 8
                                n248 = local write "选项卡控件_实验步骤2"(w209) -> ()
                                n249 = local write "选项卡控件_实验步骤3"(w209) -> ()
                                n250 = local write "选项卡控件_实验步骤1"(w209) -> ()
                                }
                              }
                              n251 = Wait (ms)(milliseconds to wait=u32 150 ("等待时间（毫秒）")) -> ()  [unwired: 1 out]
                            }
                            n252 = local write "当前放射源"(w202) -> ()
                            n253 = local write "放射源"(w202) -> ()
                          }
                        }
                        n254 = local write "按钮_放置放射源"(w191) -> ()
                        n255 = local write "按钮_放置放射源2"(w191) -> ()
                        n256 = local write "是否放置放射源"(w191) -> ()
                      }
                    }
                  }
                  frame True {
                    w210 = TRUE ("按钮_放置放射源")
                    n257 = local write "按钮_放置放射源"(w210) -> ()
                    n258 = local write "按钮_放置放射源2"(w210) -> ()
                    n259 = One Button Dialog(message="吸收片忘了取下来了" ("消息")) -> ()  [unwired: 1 in, 1 out]
                  }
                }
              }
              frame #1 {
                n260 = call <vilib>:"Unset Busy.vi"() -> ()  [unwired: 11 in, 1 out]
              }
            }
            n261 = local read "选项卡_实验内容"() -> (w154:T1)
            n262 = Equal?(x=w154, y=1) -> ()  [unwired: 1 out]
          }
          event "按钮_开始测量2": Value Change {
            n263 = event-data() -> ()  [unwired: 1 in, 6 out]
            n264 = local read "是否放置放射源"() -> (w212:bool)
            n265 = case shown="真" w212 {
              frame False {
                n266 = One Button Dialog(message="还没放放射源，会没有信号的" ("消息")) -> ()  [unwired: 1 in, 1 out]
              }
              frame True {
                n267 = local read "是否真空"() -> (w215:bool)
                n268 = case shown="真" w215 {
                  frame False {
                    n269 = One Button Dialog(message="还没抽真空，测出来的数据不准确的" ("消息")) -> ()  [unwired: 1 in, 1 out]
                  }
                  frame True {
                    n270 = local read "电压表 2"() -> (w219:i32)
                    n271 = Equal?(x=w219, y=120) -> (x = y?=w217:bool)
                    n272 = case shown="真" w217 {
                      frame False {
                        n273 = One Button Dialog(message="探测器的偏压还不是最理想的电压值" ("消息")) -> ()  [unwired: 1 in, 1 out]
                      }
                      frame True {
                        n274 = flat-sequence {
                          frame #0 {
                            w235 = "120V"
                            n275 = Current VI's Path() -> (path=w222:path)
                            n276 = call <vilib>:"Set Busy.vi"() -> ()  [unwired: 10 in, 2 out]
                            n277 = local read "放射源2"() -> (w238:string)
                            n278 = call "路径转换.vi"("input path"=w222) -> ("output path"=w223:path)
                            n279 = Strip Path(path=w223) -> (stripped path=w246:path)  [unwired: 1 out]
                            n280 = Build Path(base path=w246, name or relative path="data") -> (appended path=w247:path)
                            n281 = Concatenate Strings(w235, w238, "high.txt") -> (w240:string)
                            n282 = Concatenate Strings(w235, w238, "low.txt") -> (w236:string)
                            n283 = Build Path(base path=w247, name or relative path=w240) -> (appended path=w245:path)
                            n284 = Build Path(base path=w247, name or relative path=w236) -> (appended path=w244:path)
                            n285 = call "Find_VISA.vi"() -> ("错误输出"=w242:errorcluster, "虚拟放射源VISA"=w243:string)  [unwired: 3 in, 1 out]
                            n286 = call "虚拟放射源能谱设置.vi"("错误输入（无错误）"=w242, "低位数据路径"=w244, "高位数据路径"=w245, "VISA资源名称"=w243) -> ("错误输出"=w228:errorcluster, "VISA资源名称输出"=w229:refnum<visa-resource-name>)
                            n287 = local read "是否放置放射源"() -> (w234:bool)
                            n288 = local read "偏压输入指示 2"() -> (w233:bool)
                            n289 = local read "按钮_抽取真空"() -> (w231:bool)
                            n290 = And(x=w234, y=w233) -> (x .and. y?=w232:bool)
                            n291 = local read "放大倍数"() -> (w224:dbl)
                            n292 = And(x=w232, y=w231) -> (x .and. y?=w221:bool)
                            n293 = call "虚拟放射源设置.vi"("信号输出"=w221, "放大倍数"=w224, "错误输入（无错误）"=w228, "最小时间间隔"=u16 20, "计数率"=58, "VISA资源名称"=w229) -> ("错误输出"=w226:errorcluster, "VISA资源名称输出"=w225:refnum<visa-resource-name>)
                            n294 = local write "信号输出"(w221) -> ()
                            n295 = VISA Close(VISA resource name=w225, error in (no error)=w226) -> ()  [unwired: 1 out]
                          }
                          frame #1 {
                            n296 = call <vilib>:"Unset Busy.vi"() -> ()  [unwired: 11 in, 1 out]
                            n297 = One Button Dialog(message="电压改变完成，放射源放置完成，可以打开多道分析仪测量") -> ()  [unwired: 1 in, 1 out]
                          }
                        }
                      }
                    }
                  }
                }
              }
            }
          }
          event "按钮_开始测量3": Value Change {
            n298 = event-data() -> ()  [unwired: 1 in, 6 out]
            n299 = local read "是否放置放射源"() -> (w249:bool)
            n300 = case shown="真" w249 {
              frame False {
                n301 = One Button Dialog(message="还没放放射源，会没有信号的" ("消息")) -> ()  [unwired: 1 in, 1 out]
              }
              frame True {
                n302 = local read "是否真空"() -> (w252:bool)
                n303 = case shown="真" w252 {
                  frame False {
                    n304 = One Button Dialog(message="还没抽真空，测出来的数据不准确的" ("消息")) -> ()  [unwired: 1 in, 1 out]
                  }
                  frame True {
                    n305 = local read "是否放置吸收片"() -> (w254:bool)
                    n306 = case shown="真" w254 {
                      frame False {
                        n307 = One Button Dialog(message="还没放吸收片，这样测是没有意义的" ("消息")) -> ()  [unwired: 1 in, 1 out]
                      }
                      frame True {
                        n308 = local read "电压表 2"() -> (w258:i32)
                        n309 = Equal?(x=w258, y=120) -> (x = y?=w256:bool)
                        n310 = case shown="真" w256 {
                          frame False {
                            n311 = One Button Dialog(message="探测器的偏压还不是最理想的电压值" ("消息")) -> ()  [unwired: 1 in, 1 out]
                          }
                          frame True {
                            n312 = flat-sequence {
                              frame #0 {
                                w276 = "120V"
                                n313 = call <vilib>:"Set Busy.vi"() -> ()  [unwired: 10 in, 2 out]
                                n314 = local read "吸收片种类"() -> (w279:string)
                                n315 = Current VI's Path() -> (path=w262:path)
                                n316 = call "路径转换.vi"("input path"=w262) -> ("output path"=w261:path)
                                n317 = Strip Path(path=w261) -> (stripped path=w287:path)  [unwired: 1 out]
                                n318 = Build Path(base path=w287, name or relative path="data") -> (appended path=w288:path)
                                n319 = Concatenate Strings(w276, w279, "high.txt") -> (w283:string)
                                n320 = Concatenate Strings(w276, w279, "low.txt") -> (w280:string)
                                n321 = Build Path(base path=w288, name or relative path=w283) -> (appended path=w286:path)
                                n322 = Build Path(base path=w288, name or relative path=w280) -> (appended path=w285:path)
                                n323 = call "Find_VISA.vi"() -> ("错误输出"=w277:errorcluster, "虚拟放射源VISA"=w278:string)  [unwired: 3 in, 1 out]
                                n324 = call "虚拟放射源能谱设置.vi"("错误输入（无错误）"=w277, "低位数据路径"=w285, "高位数据路径"=w286, "VISA资源名称"=w278) -> ("错误输出"=w268:errorcluster, "VISA资源名称输出"=w269:refnum<visa-resource-name>)
                                n325 = local read "是否放置放射源"() -> (w273:bool)
                                n326 = local read "偏压输入指示 3"() -> (w274:bool)
                                n327 = local read "是否真空"() -> (w272:bool)
                                n328 = local read "是否放置吸收片"() -> (w275:bool)
                                n329 = And(x=w273, y=w272) -> (x .and. y?=w271:bool)
                                n330 = And(x=w275, y=w274) -> (x .and. y?=w270:bool)
                                n331 = local read "放大倍数"() -> (w263:dbl)
                                n332 = And(x=w270, y=w271) -> (x .and. y?=w260:bool)
                                n333 = call "虚拟放射源设置.vi"("信号输出"=w260, "放大倍数"=w263, "错误输入（无错误）"=w268, "最小时间间隔"=u16 20, "计数率"=21, "VISA资源名称"=w269) -> ("错误输出"=w265:errorcluster, "VISA资源名称输出"=w266:refnum<visa-resource-name>)
                                n334 = local write "信号输出"(w260) -> ()
                                n335 = VISA Close(VISA resource name=w266, error in (no error)=w265) -> ()  [unwired: 1 out]
                              }
                              frame #1 {
                                n336 = call <vilib>:"Unset Busy.vi"() -> ()  [unwired: 11 in, 1 out]
                                n337 = One Button Dialog(message="电压改变完成，放射源放置完成，可以打开多道分析仪测量") -> ()  [unwired: 1 in, 1 out]
                              }
                            }
                          }
                        }
                      }
                    }
                  }
                }
              }
            }
          }
          event "按钮_恢复仪器初始状态", "按钮_恢复仪器初始状态 2", "按钮_恢复仪器初始状态 3": Value Change {
            n338 = event-data() -> ()  [unwired: 1 in, 6 out]
            n339 = flat-sequence {
              frame #0 {
                w305 = 1
                w308 = T3."Enabled" ("禁用")
                n340 = call <vilib>:"Set Busy.vi"() -> ()  [unwired: 10 in, 2 out]
                n341 = local write "是否放置放射源"(FALSE ("是否放置放射源")) -> ()
                n342 = local write "是否真空"(FALSE ("是否真空")) -> ()
                n343 = local write "是否放置吸收片"(FALSE ("是否放置吸收片")) -> ()
                n344 = local write "按钮_放置放射源"(FALSE ("按钮_放置放射源")) -> ()
                n345 = local write "信号输出指示 3"(FALSE ("信号输出指示 3")) -> ()
                n346 = local write "按钮_放置放射源2"(FALSE ("按钮_放置放射源2")) -> ()
                n347 = local write "偏压输入指示"(FALSE ("偏压输入指示")) -> ()
                n348 = local write "偏压输入指示 2"(FALSE ("偏压输入指示 2")) -> ()
                n349 = local write "偏压输入指示 3"(FALSE ("偏压输入指示 3")) -> ()
                n350 = local write "信号输出指示 2"(FALSE ("信号输出指示 2")) -> ()
                n351 = local write "信号输出指示"(FALSE ("信号输出指示")) -> ()
                n352 = local write "按钮_抽取真空 2"(FALSE ("按钮_抽取真空 2")) -> ()
                n353 = local write "按钮_抽取真空 3"(FALSE ("按钮_抽取真空 3")) -> ()
                n354 = local write "按钮_抽取真空"(FALSE ("按钮_抽取真空")) -> ()
                n355 = local write "选项卡控件_实验步骤3"(w305) -> ()
                n356 = property on="放射源2" class="CmbBox"("DisabledEnum"=w308) -> ()  [unwired: 2 in, 2 out]
                n357 = property on="吸收片种类" class="CmbBox"("DisabledEnum"=w308) -> ()  [unwired: 2 in, 2 out]
                n358 = local write "选项卡控件_实验步骤1"(w305) -> ()
                n359 = local write "放射源2"("241Am" ("放射源2")) -> ()
                n360 = local write "选项卡控件_实验步骤2"(w305) -> ()
                n361 = local write "吸收片种类"("Al吸收片" ("吸收片种类")) -> ()
                n362 = local write "电压表"(0 ("电压表")) -> ()
                n363 = local write "电压表 2"(0 ("电压表 2")) -> ()
                n364 = local write "电压表 3"(0 ("电压表 3")) -> ()
                n365 = call "Find_VISA.vi"() -> ("错误输出"=w296:errorcluster, "虚拟放射源VISA"=w297:string)  [unwired: 3 in, 1 out]
                n366 = local write "信号输出"(FALSE ("信号输出")) -> ()
                n367 = call "信号输出使能.vi"("VISA资源名称"=w297, "信号输出"=FALSE, "错误输入（无错误）"=w296) -> ("元素 2"=w295:string, "错误输出 2"=w294:errorcluster)  [unwired: 11 in]
                n368 = call "吸收概率设置.vi"("错误输入（无错误）"=w294, "衰减"=u16 1, "VISA资源名称"=w295) -> ("错误输出"=w292:errorcluster, "VISA资源名称输出"=w293:refnum<visa-resource-name>)
                n369 = VISA Close(VISA resource name=w293, error in (no error)=w292) -> ()  [unwired: 1 out]
              }
              frame #1 {
                n370 = call <vilib>:"Unset Busy.vi"() -> ()  [unwired: 11 in, 1 out]
              }
            }
          }
          event "按钮_抽取真空", "按钮_抽取真空 2", "按钮_抽取真空 3": Value Change {
            n371 = event-data() -> ()  [unwired: 1 in, 6 out]
            n372 = flat-sequence {
              frame #0 {
                n373 = local read "是否放置放射源"() -> (w322:bool)
                n374 = call <vilib>:"Set Busy.vi"() -> ()  [unwired: 10 in, 2 out]
                n375 = case shown="真" w322 {
                  frame False {
                    w323 = FALSE ("按钮_抽取真空")
                    n376 = local write "按钮_抽取真空"(w323) -> ()
                    n377 = local write "按钮_抽取真空 2"(w323) -> ()
                    n378 = One Button Dialog(message="还没有放置放射源，抽真空有意义吗？" ("消息")) -> ()  [unwired: 1 in, 1 out]
                  }
                  frame True {
                    n379 = local read "是否放置吸收片"() -> (w325:bool)
                    n380 = case shown="真" w325 {
                      frame False {
                        n381 = local read "是否真空"() -> (w326:bool)
                        n382 = case shown="真" w326 {
                          frame False {
                            w327 = TRUE ("按钮_抽取真空")
                            n383 = local read "当前放射源"() -> (w328:string)
                            n384 = Equal?(x=w328, y="241Am") -> (x = y?=w330:bool)
                            n385 = local read "按钮_提示"() -> (w332:bool)
                            n386 = case shown="假" w330 {
                              frame False {
                                n387 = for {
                                N: 10 -> [_]
                                i -> [w335]
                                n388 = Quotient & Remainder(x=w335, y=2) -> (x-y*floor(x/y)=w336:i32)  [unwired: 1 out]
                                n389 = case shown="1" w336 {
                                frame 0, Default {
                                w338 = 8
                                n390 = local write "选项卡控件_实验步骤2"(w338) -> ()
                                n391 = local write "选项卡控件_实验步骤1"(w338) -> ()
                                n392 = local write "选项卡控件_实验步骤3"(w338) -> ()
                                }
                                frame 1 {
                                w339 = 4
                                n393 = local write "选项卡控件_实验步骤2"(w339) -> ()
                                n394 = local write "选项卡控件_实验步骤3"(w339) -> ()
                                n395 = local write "选项卡控件_实验步骤1"(w339) -> ()
                                }
                                }
                                n396 = Wait (ms)(milliseconds to wait=u32 150 ("等待时间（毫秒）")) -> ()  [unwired: 1 out]
                                }
                              }
                              frame True {
                                n397 = for {
                                N: 10 -> [_]
                                i -> [w344]
                                n398 = Quotient & Remainder(x=w344, y=2) -> (x-y*floor(x/y)=w342:i32)  [unwired: 1 out]
                                n399 = Wait (ms)(milliseconds to wait=u32 150 ("等待时间（毫秒）")) -> ()  [unwired: 1 out]
                                n400 = case shown="1" w342 {
                                frame 0, Default {
                                w345 = 2
                                n401 = local write "选项卡控件_实验步骤1"(w345) -> ()
                                n402 = local write "选项卡控件_实验步骤3"(w345) -> ()
                                n403 = local write "选项卡控件_实验步骤2"(w345) -> ()
                                }
                                frame 1 {
                                w346 = 3
                                n404 = local write "选项卡控件_实验步骤3"(w346) -> ()
                                n405 = local write "选项卡控件_实验步骤1"(w346) -> ()
                                n406 = local write "选项卡控件_实验步骤2"(w346) -> ()
                                }
                                }
                                }
                              }
                            }
                            n407 = local write "是否真空"(TRUE) -> ()
                            n408 = case shown="假" w332 {
                              frame False {
                                n409 = local write "选项卡控件_操作步骤1"(3) -> ()
                              }
                              frame True {
                                n410 = local write "选项卡控件_操作步骤1"(2) -> ()
                              }
                            }
                            n411 = local write "按钮_抽取真空"(w327) -> ()
                            n412 = local write "按钮_抽取真空 3"(w327) -> ()
                            n413 = local write "按钮_抽取真空 2"(w327) -> ()
                          }
                          frame True {
                            w355 = FALSE ("按钮_抽取真空 2")
                            w349 = FALSE
                            n414 = local read "当前放射源"() -> (w356:string)
                            n415 = call "Find_VISA.vi"() -> ("错误输出"=w352:errorcluster, "虚拟放射源VISA"=w351:string)  [unwired: 3 in, 1 out]
                            n416 = Equal?(x=w356, y="241Am") -> (x = y?=w357:bool)
                            n417 = local read "按钮_提示"() -> (w359:bool)
                            n418 = call "信号输出使能.vi"("VISA资源名称"=w351, "信号输出"=FALSE, "错误输入（无错误）"=w352) -> ("元素 2"=w353:string, "错误输出 2"=w354:errorcluster)  [unwired: 11 in]
                            n419 = case shown="假" w357 {
                              frame False {
                                n420 = for {
                                N: 10 -> [_]
                                i -> [w362]
                                n421 = Quotient & Remainder(x=w362, y=2) -> (x-y*floor(x/y)=w363:i32)  [unwired: 1 out]
                                n422 = case shown="0, 默认" w363 {
                                frame 0, Default {
                                w365 = 4
                                n423 = local write "选项卡控件_实验步骤2"(w365) -> ()
                                n424 = local write "选项卡控件_实验步骤3"(w365) -> ()
                                n425 = local write "选项卡控件_实验步骤1"(w365) -> ()
                                }
                                frame 1 {
                                w366 = 8
                                n426 = local write "选项卡控件_实验步骤3"(w366) -> ()
                                n427 = local write "选项卡控件_实验步骤1"(w366) -> ()
                                n428 = local write "选项卡控件_实验步骤2"(w366) -> ()
                                }
                                }
                                n429 = Wait (ms)(milliseconds to wait=u32 150 ("等待时间（毫秒）")) -> ()  [unwired: 1 out]
                                }
                              }
                              frame True {
                                n430 = for {
                                N: 10 -> [_]
                                i -> [w371]
                                n431 = Quotient & Remainder(x=w371, y=2) -> (x-y*floor(x/y)=w369:i32)  [unwired: 1 out]
                                n432 = Wait (ms)(milliseconds to wait=u32 150 ("等待时间（毫秒）")) -> ()  [unwired: 1 out]
                                n433 = case shown="1" w369 {
                                frame 0, Default {
                                w372 = 3
                                n434 = local write "选项卡控件_实验步骤3"(w372) -> ()
                                n435 = local write "选项卡控件_实验步骤2"(w372) -> ()
                                n436 = local write "选项卡控件_实验步骤1"(w372) -> ()
                                }
                                frame 1 {
                                w373 = 2
                                n437 = local write "选项卡控件_实验步骤1"(w373) -> ()
                                n438 = local write "选项卡控件_实验步骤3"(w373) -> ()
                                n439 = local write "选项卡控件_实验步骤2"(w373) -> ()
                                }
                                }
                                }
                              }
                            }
                            n440 = VISA Close(VISA resource name=w353, error in (no error)=w354) -> ()  [unwired: 1 out]
                            n441 = case shown="假" w359 {
                              frame False {
                                n442 = local write "选项卡控件_操作步骤1"(3) -> ()
                              }
                              frame True {
                                n443 = local write "选项卡控件_操作步骤1"(1) -> ()
                              }
                            }
                            n444 = local write "是否真空"(w349) -> ()
                            n445 = local write "信号输出"(w349) -> ()
                            n446 = local write "按钮_抽取真空"(w355) -> ()
                            n447 = local write "按钮_抽取真空 2"(w355) -> ()
                            n448 = local write "按钮_抽取真空 3"(w355) -> ()
                          }
                        }
                      }
                      frame True {
                        n449 = local read "吸收片种类"() -> (w378:string)
                        n450 = Equal?(x=w378, y="Al吸收片") -> (x = y?=w376:bool)
                        n451 = case shown="真" w376 {
                          frame False {
                            n452 = local read "是否真空"() -> (w379:bool)
                            n453 = case shown="真" w379 {
                              frame False {
                                w381 = TRUE ("按钮_抽取真空")
                                n454 = for {
                                N: 10 -> [_]
                                i -> [w385]
                                n455 = Quotient & Remainder(x=w385, y=2) -> (x-y*floor(x/y)=w386:i32)  [unwired: 1 out]
                                n456 = case shown="1" w386 {
                                frame 0, Default {
                                w388 = 10
                                n457 = local write "选项卡控件_实验步骤2"(w388) -> ()
                                n458 = local write "选项卡控件_实验步骤3"(w388) -> ()
                                n459 = local write "选项卡控件_实验步骤1"(w388) -> ()
                                }
                                frame 1 {
                                w389 = 6
                                n460 = local write "选项卡控件_实验步骤2"(w389) -> ()
                                n461 = local write "选项卡控件_实验步骤3"(w389) -> ()
                                n462 = local write "选项卡控件_实验步骤1"(w389) -> ()
                                }
                                }
                                n463 = Wait (ms)(milliseconds to wait=u32 150 ("等待时间（毫秒）")) -> ()  [unwired: 1 out]
                                }
                                n464 = local write "是否真空"(TRUE ("是否真空")) -> ()
                                n465 = property on="吸收片种类" class="CmbBox"("DisabledEnum"=T3."Disabled and Grayed Out" ("禁用")) -> ()  [unwired: 2 in, 2 out]
                                n466 = local write "按钮_抽取真空 2"(w381) -> ()
                                n467 = local write "按钮_抽取真空 3"(w381) -> ()
                                n468 = local write "按钮_抽取真空"(w381) -> ()
                              }
                              frame True {
                                w397 = FALSE ("按钮_抽取真空")
                                w390 = FALSE ("是否真空")
                                n469 = local write "信号输出"(w390) -> ()
                                n470 = local write "是否真空"(w390) -> ()
                                n471 = property on="吸收片种类" class="CmbBox"("DisabledEnum"=T3."Enabled" ("禁用")) -> ()  [unwired: 2 in, 2 out]
                                n472 = for {
                                N: 10 -> [_]
                                i -> [w400]
                                n473 = Quotient & Remainder(x=w400, y=2) -> (x-y*floor(x/y)=w401:i32)  [unwired: 1 out]
                                n474 = case shown="1" w401 {
                                frame 0, Default {
                                w403 = 6
                                n475 = local write "选项卡控件_实验步骤3"(w403) -> ()
                                n476 = local write "选项卡控件_实验步骤2"(w403) -> ()
                                n477 = local write "选项卡控件_实验步骤1"(w403) -> ()
                                }
                                frame 1 {
                                w404 = 10
                                n478 = local write "选项卡控件_实验步骤2"(w404) -> ()
                                n479 = local write "选项卡控件_实验步骤3"(w404) -> ()
                                n480 = local write "选项卡控件_实验步骤1"(w404) -> ()
                                }
                                }
                                n481 = Wait (ms)(milliseconds to wait=u32 150 ("等待时间（毫秒）")) -> ()  [unwired: 1 out]
                                }
                                n482 = local write "按钮_抽取真空 2"(w397) -> ()
                                n483 = local write "按钮_抽取真空"(w397) -> ()
                                n484 = local write "按钮_抽取真空 3"(w397) -> ()
                                n485 = call "Find_VISA.vi"() -> ("错误输出"=w393:errorcluster, "虚拟放射源VISA"=w392:string)  [unwired: 3 in, 1 out]
                                n486 = call "信号输出使能.vi"("VISA资源名称"=w392, "信号输出"=FALSE, "错误输入（无错误）"=w393) -> ("元素 2"=w394:string, "错误输出 2"=w395:errorcluster)  [unwired: 11 in]
                                n487 = VISA Close(VISA resource name=w394, error in (no error)=w395) -> ()  [unwired: 1 out]
                              }
                            }
                          }
                          frame True {
                            n488 = local read "是否真空"() -> (w405:bool)
                            n489 = case shown="真" w405 {
                              frame False {
                                w407 = TRUE ("按钮_抽取真空")
                                n490 = for {
                                N: 10 -> [_]
                                i -> [w411]
                                n491 = Quotient & Remainder(x=w411, y=2) -> (x-y*floor(x/y)=w412:i32)  [unwired: 1 out]
                                n492 = case shown="0, 默认" w412 {
                                frame 0, Default {
                                w414 = 9
                                n493 = local write "选项卡控件_实验步骤3"(w414) -> ()
                                n494 = local write "选项卡控件_实验步骤2"(w414) -> ()
                                n495 = local write "选项卡控件_实验步骤1"(w414) -> ()
                                }
                                frame 1 {
                                w415 = 5
                                n496 = local write "选项卡控件_实验步骤3"(w415) -> ()
                                n497 = local write "选项卡控件_实验步骤2"(w415) -> ()
                                n498 = local write "选项卡控件_实验步骤1"(w415) -> ()
                                }
                                }
                                n499 = Wait (ms)(milliseconds to wait=u32 150 ("等待时间（毫秒）")) -> ()  [unwired: 1 out]
                                }
                                n500 = local write "是否真空"(TRUE ("是否真空")) -> ()
                                n501 = property on="吸收片种类" class="CmbBox"("DisabledEnum"=T3."Disabled and Grayed Out" ("禁用")) -> ()  [unwired: 2 in, 2 out]
                                n502 = local write "按钮_抽取真空"(w407) -> ()
                                n503 = local write "按钮_抽取真空 2"(w407) -> ()
                                n504 = local write "按钮_抽取真空 3"(w407) -> ()
                              }
                              frame True {
                                w423 = FALSE ("按钮_抽取真空")
                                w416 = FALSE ("是否真空")
                                n505 = for {
                                N: 10 -> [_]
                                i -> [w426]
                                n506 = Quotient & Remainder(x=w426, y=2) -> (x-y*floor(x/y)=w427:i32)  [unwired: 1 out]
                                n507 = case shown="0, 默认" w427 {
                                frame 0, Default {
                                w429 = 5
                                n508 = local write "选项卡控件_实验步骤2"(w429) -> ()
                                n509 = local write "选项卡控件_实验步骤3"(w429) -> ()
                                n510 = local write "选项卡控件_实验步骤1"(w429) -> ()
                                }
                                frame 1 {
                                w430 = 9
                                n511 = local write "选项卡控件_实验步骤2"(w430) -> ()
                                n512 = local write "选项卡控件_实验步骤3"(w430) -> ()
                                n513 = local write "选项卡控件_实验步骤1"(w430) -> ()
                                }
                                }
                                n514 = Wait (ms)(milliseconds to wait=u32 150 ("等待时间（毫秒）")) -> ()  [unwired: 1 out]
                                }
                                n515 = local write "是否真空"(w416) -> ()
                                n516 = local write "信号输出"(w416) -> ()
                                n517 = call "Find_VISA.vi"() -> ("错误输出"=w419:errorcluster, "虚拟放射源VISA"=w418:string)  [unwired: 3 in, 1 out]
                                n518 = call "信号输出使能.vi"("VISA资源名称"=w418, "信号输出"=FALSE, "错误输入（无错误）"=w419) -> ("元素 2"=w420:string, "错误输出 2"=w421:errorcluster)  [unwired: 11 in]
                                n519 = VISA Close(VISA resource name=w420, error in (no error)=w421) -> ()  [unwired: 1 out]
                                n520 = local write "按钮_抽取真空"(w423) -> ()
                                n521 = local write "按钮_抽取真空 2"(w423) -> ()
                                n522 = local write "按钮_抽取真空 3"(w423) -> ()
                                n523 = property on="吸收片种类" class="CmbBox"("DisabledEnum"=T3."Enabled" ("禁用")) -> ()  [unwired: 2 in, 2 out]
                              }
                            }
                          }
                        }
                      }
                    }
                  }
                }
              }
              frame #1 {
                n524 = call <vilib>:"Unset Busy.vi"() -> ()  [unwired: 11 in, 1 out]
              }
            }
          }
        }
      }
      frame "完成" {
      }
    }
  }
  n525 = flat-sequence {
    tunnel: w2 -> [w433]
    tunnel: [w433] -> w1
    frame #0 {
      n526 = local write "退出"(FALSE) -> ()
    }
  }
  n527 = while {
    tunnel: w1 -> [_]
    stop <- w437 stop-if-true
    n528 = local read "信号输出"() -> (w438:bool)
    n529 = case shown="真" w438 {
      frame False {
        w439 = FALSE
        n530 = local write "信号输出指示"(w439) -> ()
        n531 = local write "信号输出指示 2"(w439) -> ()
        n532 = Wait (ms)(milliseconds to wait=u32 300 ("等待时间（毫秒）")) -> ()  [unwired: 1 out]
        n533 = local write "信号输出指示 3"(w439) -> ()
      }
      frame True {
        n534 = local read "信号输出指示"() -> (w446:bool)
        n535 = local read "信号输出指示 2"() -> (w444:bool)
        n536 = local read "信号输出指示 3"() -> (w442:bool)
        n537 = Not(x=w446) -> (.not. x?=w445:bool)
        n538 = Not(x=w444) -> (.not. x?=w443:bool)
        n539 = Not(x=w442) -> (.not. x?=w441:bool)
        n540 = Wait (ms)(milliseconds to wait=u32 300 ("等待时间（毫秒）")) -> ()  [unwired: 1 out]
        n541 = local write "信号输出指示 2"(w443) -> ()
        n542 = local write "信号输出指示 3"(w441) -> ()
        n543 = local write "信号输出指示"(w445) -> ()
      }
    }
    n544 = local read "电压表"() -> (w436:i32)
    n545 = Greater Than 0?(x=w436) -> (x > 0?=w435:bool)
    n546 = local write "偏压输入指示 2"(w435) -> ()
    n547 = local write "偏压输入指示"(w435) -> ()
    n548 = local write "偏压输入指示 3"(w435) -> ()
    n549 = local read "退出"() -> (w437:bool)
  }
